vi "Test - SubVI Multiply.vi"(10 "Array":dbl[](array[numeric])) -> (2 "Numeric":dbl)   [LabVIEW 2019]
doc: "This VI is used by the Creating New VI From Scratch.vi and Creating New VI From Template.vi examples."
panel:
  # "Select Help>>Show Context Help and move the cursor over the VI icon to display help for this VI."
  # "This VI is used by the Creating New VI From Scratch.vi and Creating New VI From Template.vi examples."
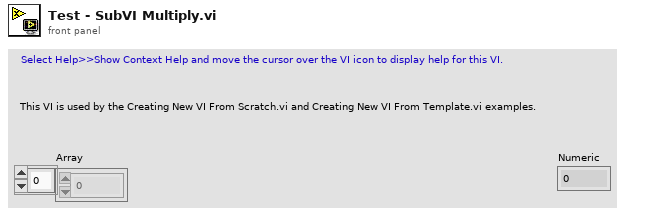
[diagram p1: front panel]
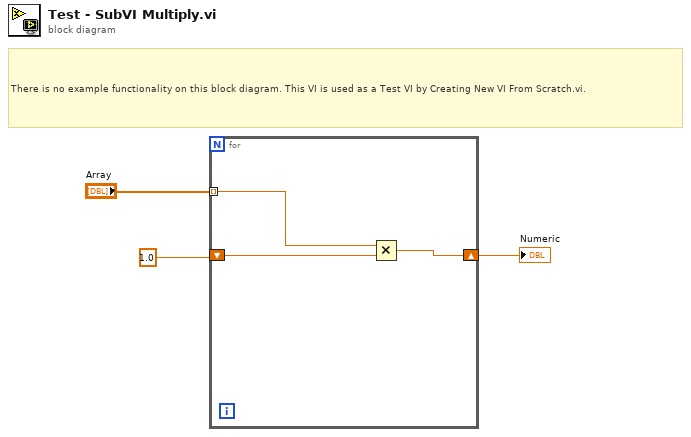
[diagram p0: block diagram]
diagram:
  # "There is no example functionality on this block diagram. This VI is used as a Test VI by Creating New VI From Scratch.vi."
  n1 = for {
    tunnel: "Array" -> [w5] mode=indexing
    shift-right: [w4] -> w1
    shift-left: 1.0 -> [w6]
    n2 = Multiply(x=w5, y=w6) -> (x*y=w4:dbl)
  }
  "Numeric" <- w1
